vi "loadSocketMDB.vi"() -> ()   [LabVIEW 2012]
uses:
  <vilib>/addons/database/Connection.llb/DB Tools Open Connec (Path).vi
  <vilib>/addons/database/Connection.llb/DB Tools Open Connec (String).vi
  <vilib>/addons/database/Connection.llb/Conn Execute.vi
  <vilib>/addons/database/Recordset.llb/Rec Fetch Recordset Data (R).vi
  <vilib>/addons/database/Recordset.llb/Rec Destroy - Connection.vi
  <vilib>/addons/database/_DB Variant To Data/Database Variant To Data.xnode
  <vilib>/addons/database/NI_Database_API.lvlib
panel:
  out "output cluster":T1
  in  "string":string="DataBase.mdb"
  out "error out 2":errorcluster
  out "recordset data":variant[][](array[variant])
  in  "Cluster":T1
  out "error out":errorcluster
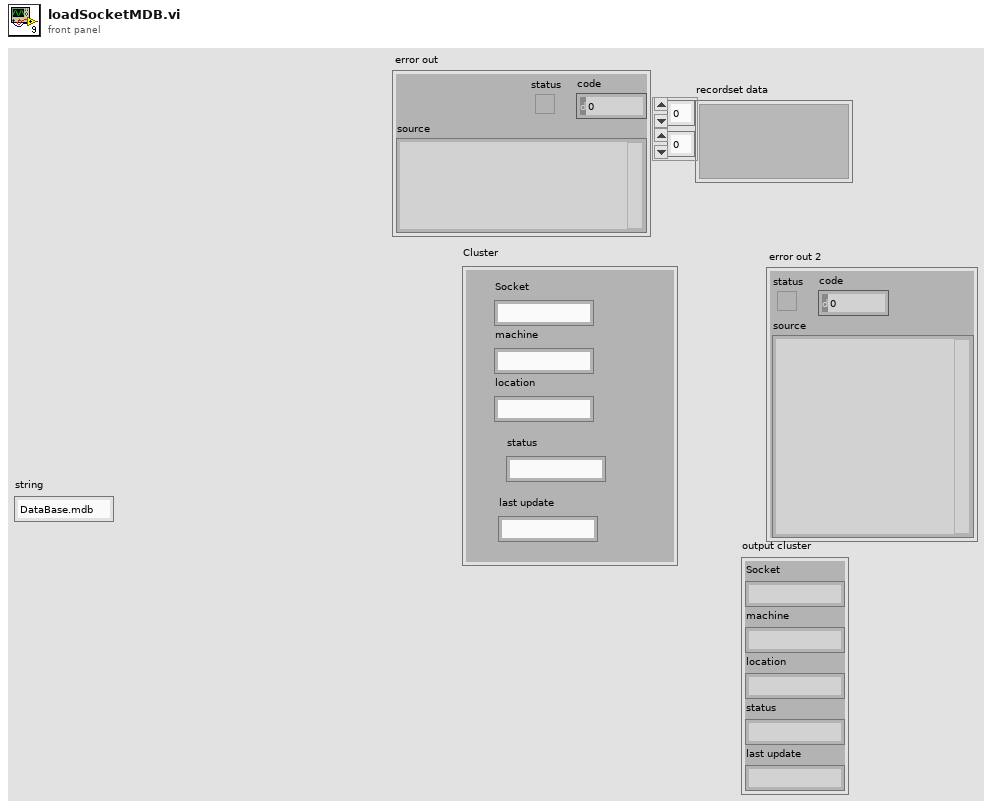
[diagram p1: front panel]
types:
  T1 = cluster{"Socket":string, "machine ":string, "location ":string, "status ":string, "last update ":string}
  T2 = typedef "NI_Database_API.lvlib/Conn ObjectReference.ctl" = refnum<k1>
  T3 = typedef "NI_Database_API.lvlib/Rec ObjectReference.ctl" = refnum<k1>
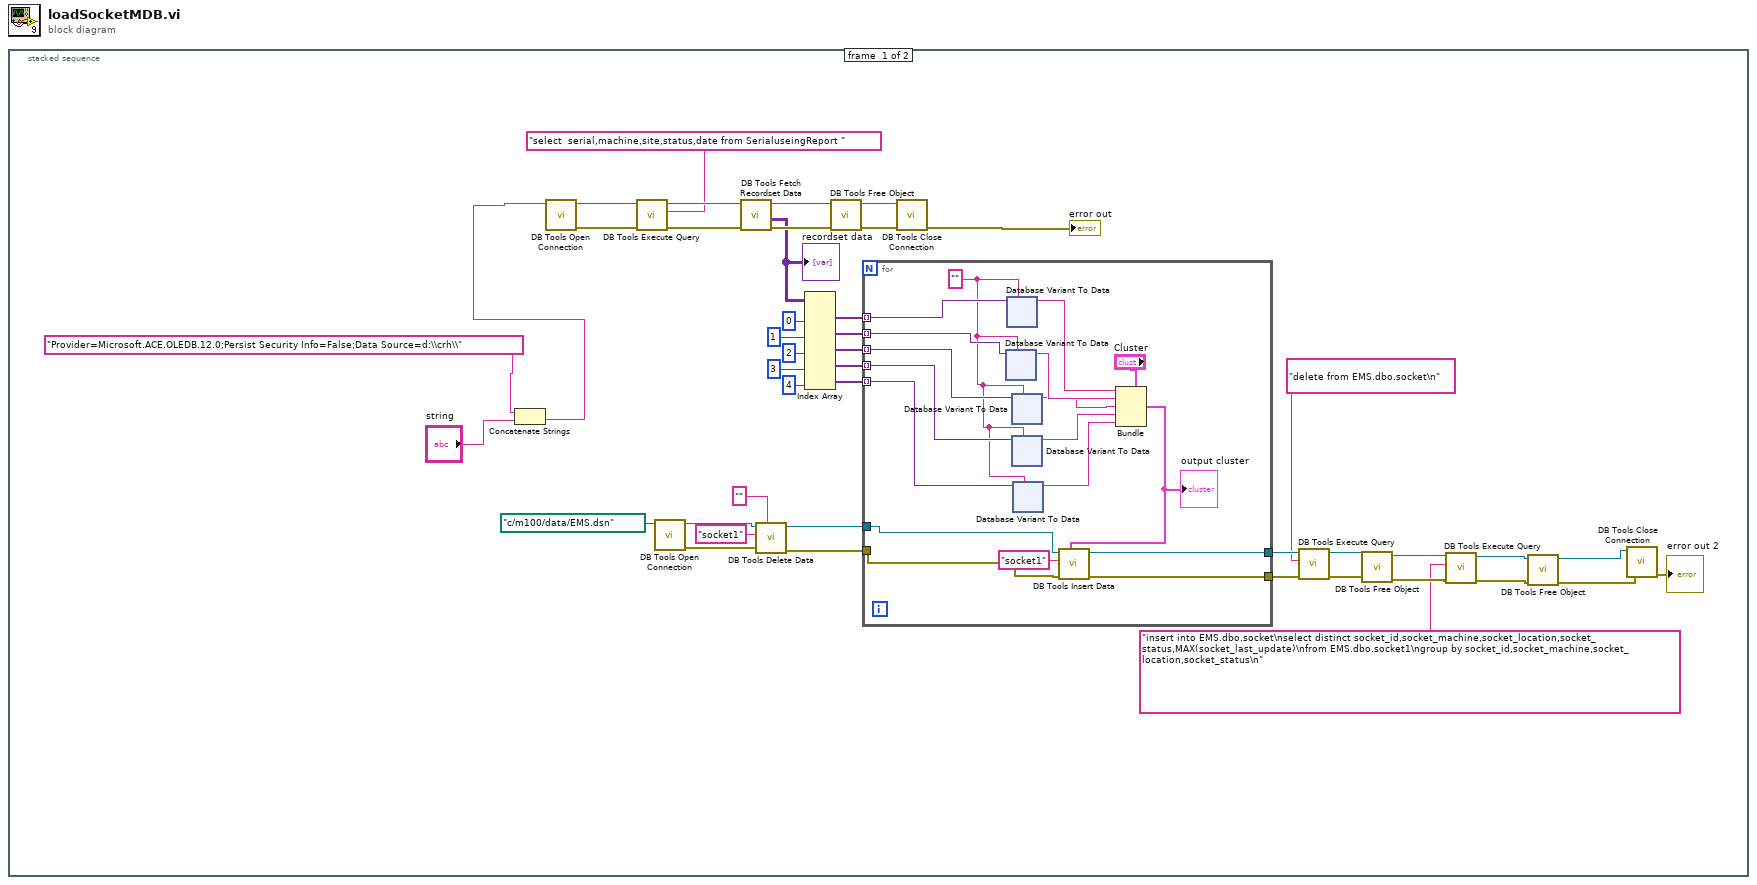
[diagram p0: block diagram]
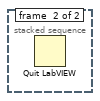
[diagram p2: hidden frame]
diagram:
  n1 = stacked-sequence {
    frame #0 {
      n2 = Concatenate Strings("Provider=Microsoft.ACE.OLEDB.12.0;Persist Security Info=False;Data Source=d:\\crh\\", "string") -> (w9:string)
      n3 = call-poly <vilib>:"DB Tools Open Connection.vi"("connection information"=w9) -> ("error out"=w40:errorcluster, "connection reference"=w44:T2)  [unwired: 7 in]
      n4 = call-poly <vilib>:"DB Tools Execute Query.vi"("error in (no error)"=w40, "SQL query"="select  serial,machine,site,status,date from SerialuseingReport ", "connection reference"=w44) -> ("error out"=w39:errorcluster, "recordset reference"=w43:T3)  [unwired: 5 in]
      n5 = call-poly <vilib>:"DB Tools Open Connection.vi"("connection information"=path "c:/m100/data/EMS.dsn") -> ("error out"=w21:errorcluster, "connection reference"=w22:T2)  [unwired: 7 in]
      n6 = call-poly <vilib>:"DB Tools Fetch Recordset Data.vi"("error in (no error)"=w39, "recordset reference"=w43) -> ("error out"=w38:errorcluster, "recordset data"=w34:variant[][], "recordset reference out"=w42:T3)  [unwired: 3 in]
      "recordset data" <- w34
      n7 = call <vilib>:"DB Tools Delete Data.vi"("condition"="", "error in (no error)"=w21, "table"="socket1", "connection reference"=w22) -> ("error out"=w19:errorcluster, "connection reference out"=w20:T2)  [unwired: 6 in]
      n8 = Index Array(array=w34, index (col) #1=0 ("disabled index (col)"), index (col) #2=1 ("index (col)"), index (col) #3=2 ("index (col)"), index (col) #4=3 ("index (col)"), index (col) #5=4 ("index (col)")) -> (element #1=w28:variant[], element #2=w27:variant[], element #3=w26:variant[], element #4=w25:variant[], element #5=w24:variant[])  [unwired: 5 in]
      n9 = call-poly <vilib>:"DB Tools Free Object.vi"("error in (no error)"=w38, "recordset reference"=w42) -> ("error out"=w37:errorcluster, "connection reference"=w41:T2)  [unwired: 8 in]
      n10 = for {
        tunnel: w28 -> [w62] mode=indexing
        tunnel: w27 -> [w61] mode=indexing
        tunnel: w26 -> [w60] mode=indexing
        tunnel: w25 -> [w59] mode=indexing
        tunnel: w24 -> [w58] mode=indexing
        tunnel: w20 -> [w50]
        tunnel: w19 -> [w49]
        tunnel: [w48] -> w13
        tunnel: [w47] -> w12
        w57 = ""
        n11 = xnode "Database Variant To Data"("database variant"=w61, "type"=w57) -> ("data"=w54:string)  [unwired: 1 in, 1 out]
        n12 = xnode "Database Variant To Data"("database variant"=w62, "type"=w57) -> ("data"=w55:string)  [unwired: 1 in, 1 out]
        n13 = xnode "Database Variant To Data"("database variant"=w60, "type"=w57) -> ("data"=w53:string)  [unwired: 1 in, 1 out]
        n14 = xnode "Database Variant To Data"("database variant"=w59, "type"=w57) -> ("data"=w52:string)  [unwired: 1 in, 1 out]
        n15 = xnode "Database Variant To Data"("database variant"=w58, "type"=w57) -> ("data"=w51:string)  [unwired: 1 in, 1 out]
        n16 = Bundle(cluster="Cluster", "Socket"=w55, "machine"=w54, "location"=w53, "status"=w52, "last update"=w51) -> (w46:T1)
        "output cluster" <- w46
        n17 = call <vilib>:"DB Tools Insert Data.vi"("data"=w46, "error in (no error)"=w49, "table"="socket1", "connection reference"=w50) -> ("error out"=w47:errorcluster, "connection reference out"=w48:T2)  [unwired: 6 in]
      }
      n18 = call <vilib>:"DB Tools Close Connection.vi"("error in (no error)"=w37, "connection reference"=w41) -> ("error out"=→"error out":errorcluster)  [unwired: 5 in]
      n19 = call-poly <vilib>:"DB Tools Execute Query.vi"("error in (no error)"=w12, "SQL query"="delete from EMS.dbo.socket\n", "connection reference"=w13) -> ("error out"=w14:errorcluster, "recordset reference"=w15:T3)  [unwired: 5 in]
      n20 = call-poly <vilib>:"DB Tools Free Object.vi"("error in (no error)"=w14, "recordset reference"=w15) -> ("error out"=w5:errorcluster, "connection reference"=w2:T2)  [unwired: 8 in]
      n21 = call-poly <vilib>:"DB Tools Execute Query.vi"("error in (no error)"=w5, "SQL query"="insert into EMS.dbo.socket\nselect distinct socket_id,socket_machine,socket_location,socket_status,MAX(socket_last_update)\nfrom EMS.dbo.socket1\ngroup by socket_id,socket_machine,socket_location,socket_status\n", "connection reference"=w2) -> ("error out"=w4:errorcluster, "recordset reference"=w7:T3)  [unwired: 5 in]
      n22 = call-poly <vilib>:"DB Tools Free Object.vi"("error in (no error)"=w4, "recordset reference"=w7) -> ("error out"=w3:errorcluster, "connection reference"=w6:T2)  [unwired: 8 in]
      n23 = call <vilib>:"DB Tools Close Connection.vi"("error in (no error)"=w3, "connection reference"=w6) -> ("error out"=→"error out 2":errorcluster)  [unwired: 5 in]
    }
    frame #1 {
      n24 = Quit LabVIEW() -> ()  [unwired: 1 in]
    }
  }
